vi "Model Initial Values - Main Page.vi"(8 "error in (no error)":errorcluster, 11 "Node Ptr":T1 format="%.0x") -> (0 "error out":errorcluster)   [LabVIEW 2011, in "Model Initial Values Custom Device.lvlib"]
uses:
  Model Initial Values Custom Device.lvlib
  <vilib>/NI Veristand/Custom Device API/Custom Device Item Ref.ctl
  <vilib>/event_ctls.llb/eventvkey.ctl
  <vilib>/NI Veristand/Custom Device API/Custom Device API.lvlib
  Model Initial Values - Global.vi
  <vilib>/NI Veristand/Custom Device Tools/Custom Device Utility Library/Custom Device Utility Library.lvlib
panel:
  in  "Models":i32[](listbox)
  in  "SHDocVw.IWebBrowser2":refnum<k7>(container)
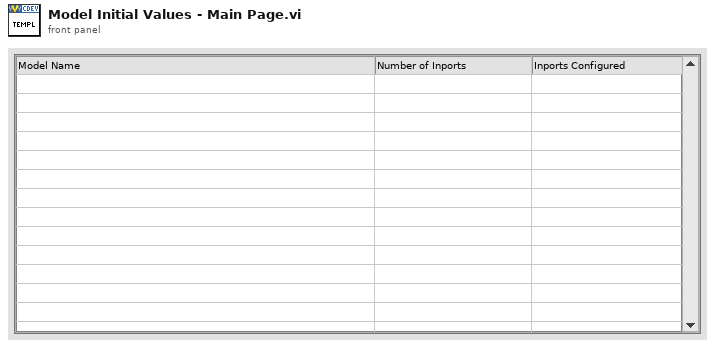
[diagram p1: front panel]
types:
  T1 = typedef "Custom Device API.lvlib/Custom Device Item Ref.ctl" = u64
  T2 = cluster{"Name":string, "Is Channel":bool, "GUID":string}
  T3 = typedef "eventvkey.ctl" = enum16{"ASCII", "Enter", "Return", "Shift", "Ctrl", "Alt", "Cmd", "Opt", "Caps", "NumLock", "Clear", "Break", "Up", "Down", "Left", "Right", "Insert", "Delete", "Home", "End", "PageUp", "PageDown", "Escape", "Help", "Pause", "ScrollLock", "F1", "F2", "F3", "F4", "F5", "F6", "F7", "F8", "F9", "F10", "F11", "F12", "F13", "F14", "F15", "F16", "F17", "F18", "F19", "F20", "F21", "F22", "F23", "F24", "Play", "VolumeUp", "VolumeDown", "Mute", "Two Byte Char"}
  T4 = typedef "Custom Device API.lvlib/Custom Device Commands.ctl" = enum16{"Default", "Item renamed", "Shutdown", "Dynamic button pressed"}
  T5 = enum16{"open", "replace", "create", "open or create", "replace or create", "replace or create with confirmation"}
  T6 = cluster{"MultipleSelection":bool, "ShowCheckBox":bool}
  T7 = typedef "Custom Device API.lvlib/Custom Device Item Info.ctl" = cluster{"Name":string, "Is Channel":bool, "GUID":string}
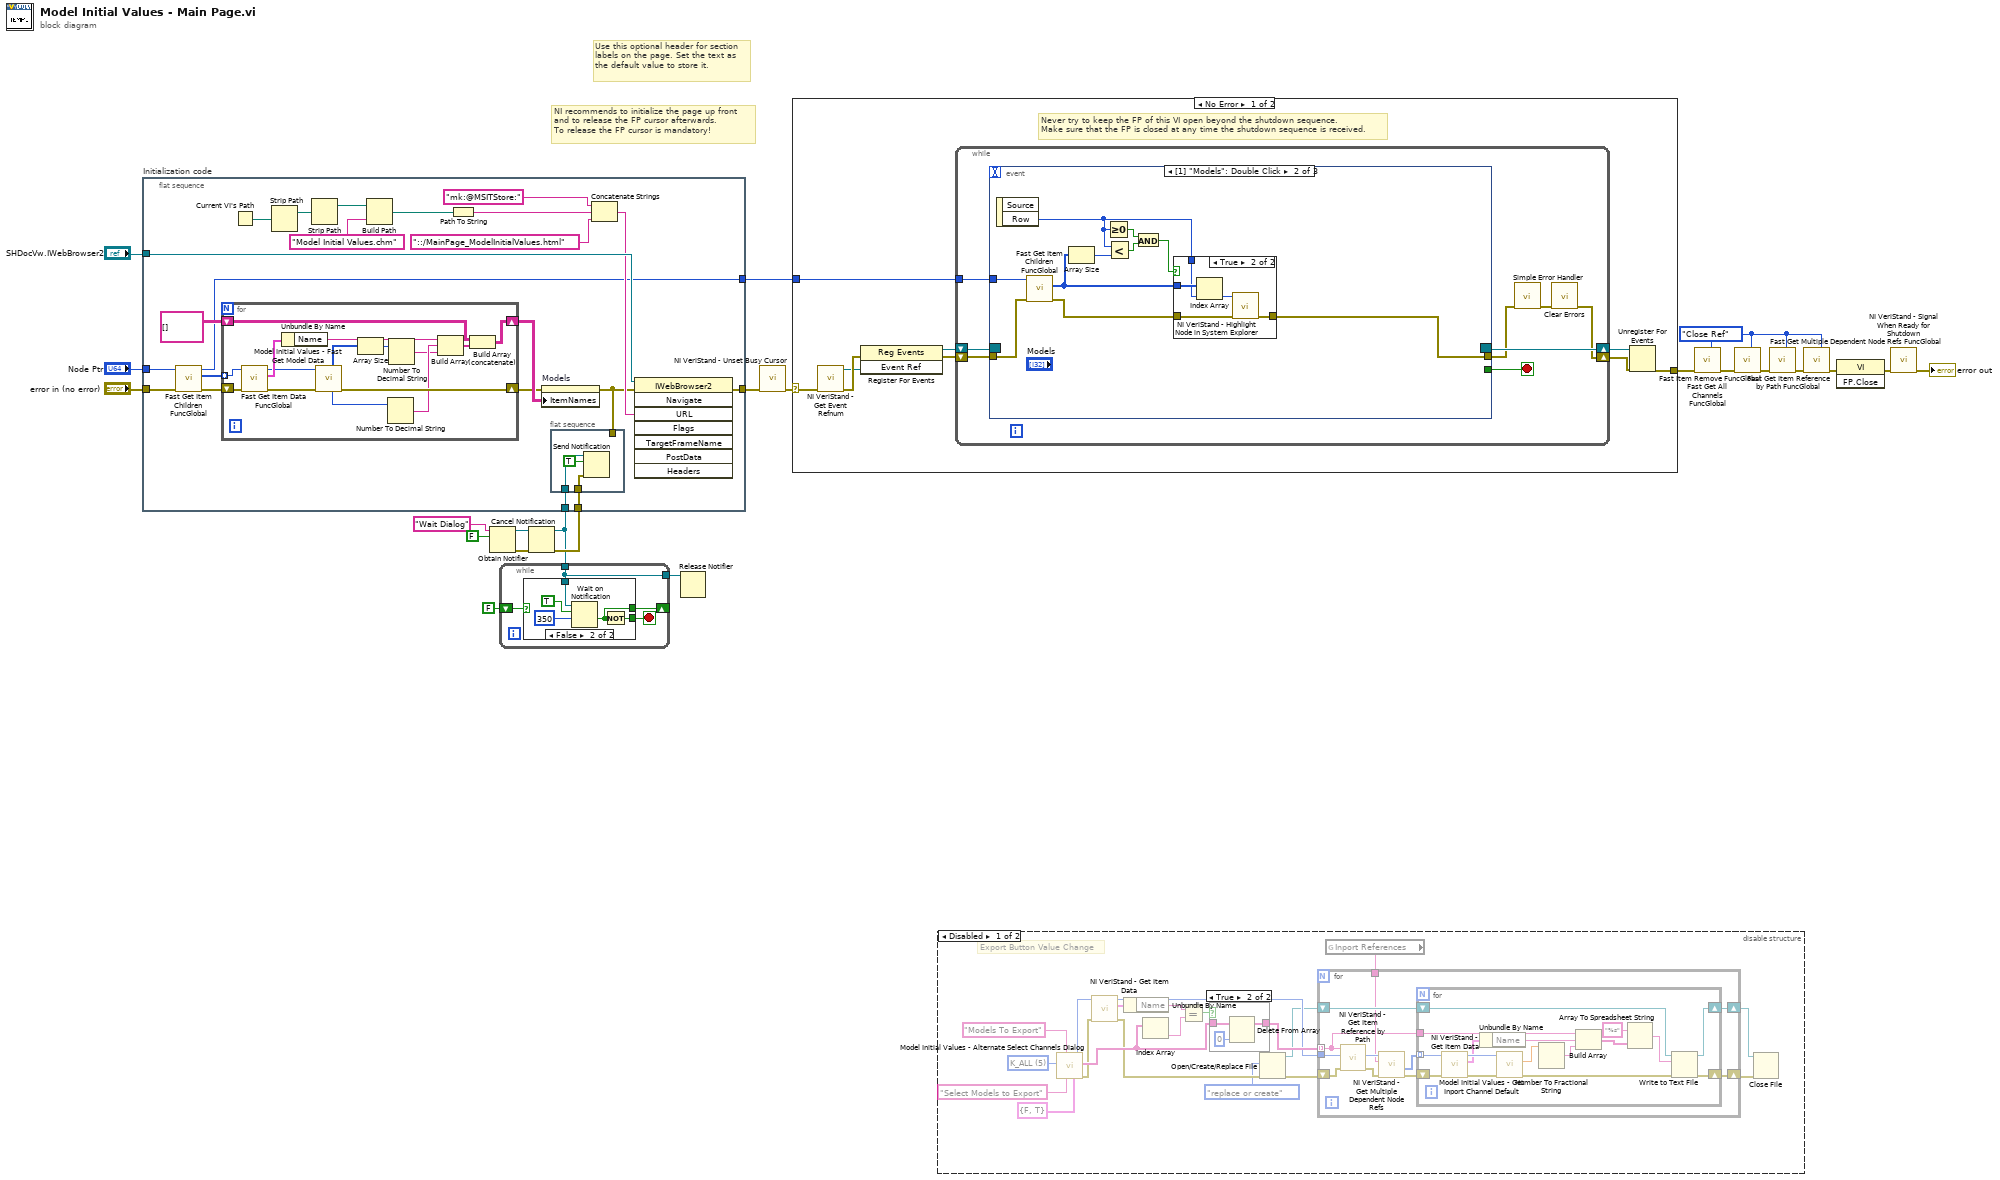
[diagram p0: block diagram]
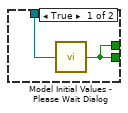
[diagram p2: hidden frame]
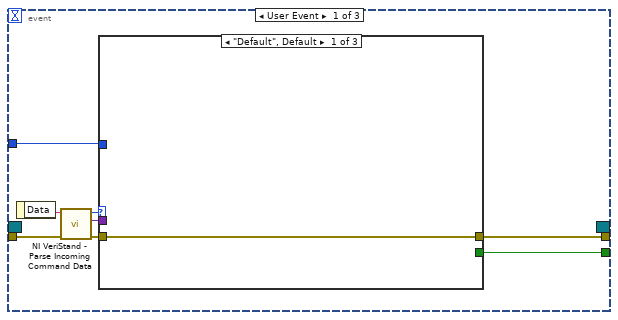
[diagram p5: hidden frame]
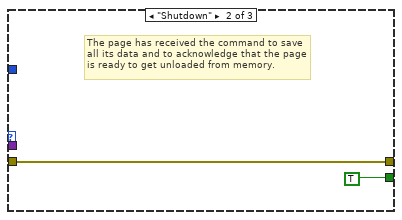
[diagram p6: hidden frame]
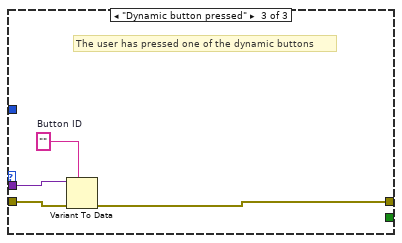
[diagram p7: hidden frame]
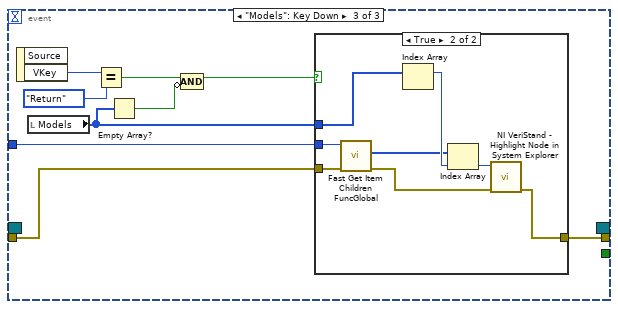
[diagram p9: hidden frame]
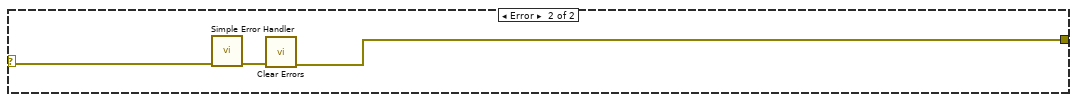
[diagram p11: hidden frame]
diagram:
  w1 = enum16{"Open or Add", "Close Ref"}."Close Ref" ("Action")
  # "Use this optional header for section labels on the page. Set the text as the default value to store it."
  # "NI recommends to initialize the page up front\nand to release the FP cursor afterwards.\nTo release the FP cursor is mandatory!"
  n1 = flat-sequence "Initialization code" {
    tunnel: "error in (no error)" -> [w24]
    tunnel: "Node Ptr" -> [w25]
    tunnel: [w43] -> w20
    tunnel: [w28] -> w17
    tunnel: "SHDocVw.IWebBrowser2" -> [w42]
    tunnel: w4 -> [w27]
    tunnel: w5 -> [w26]
    frame #0 {
      n2 = call "Fast Get Item Children FuncGlobal.vi"("error in (no error)"=w24, "Item Ref in"=w25) -> ("error out"=w30:errorcluster, "Child Refs"=w29:T1[], "Item Ref out"=w28:T1)  [unwired: 6 in, 1 out]
      n3 = for {
        tunnel: w29 -> [w58] mode=indexing
        shift-right: [w61] -> w31
        shift-left: w30 -> [w59]
        shift-right: [w62] -> w44
        shift-left: string[][] [] -> [w60]
        n4 = call "Fast Get Item Data FuncGlobal.vi"("error in (no error)"=w59, "Item Ref in"=w58) -> ("error out"=w49:errorcluster, "Item Info"=w51:T2, "Item Ref out"=w50:T1)  [unwired: 6 in, 1 out]
        n5 = Unbundle By Name(w51) -> ("Name"=w48:string)
        n6 = call "Model Initial Values - Fast Get Model Data.vi"("error in (no error)"=w49, "Local Model Ref in"=w50) -> ("error out"=w61:errorcluster, "Num Inports"=w56:i32, "Inport Refs"=w53:T1[])  [unwired: 4 in, 3 out]
        n7 = Array Size(array=w53) -> (size(s)=w54:i32)
        n8 = Number To Decimal String(number=w56) -> (decimal integer string=w55:string)  [unwired: 1 in]
        n9 = Number To Decimal String(number=w54) -> (decimal integer string=w52:string)  [unwired: 1 in]
        n10 = Build Array(w48, w55, w52) -> (w57:string[])
        n11 = Build Array (concatenate)(w60, w57) -> (w62:string[][])
      }
      n12 = Current VI's Path() -> (path=w33:path)
      n13 = Strip Path(path=w33) -> (stripped path=w34:path)  [unwired: 1 out]
      n14 = Strip Path(path=w34) -> (stripped path=w41:path)  [unwired: 1 out]
      n15 = Build Path(base path=w41, name or relative path="Model Initial Values.chm") -> (appended path=w39:path)
      n16 = Path To String(path=w39) -> (string=w38:string)
      n17 = property on="Models" class="MCListbox (strict)"(error in=w31, "ItemNames"=w44) -> (error out=w23:errorcluster)  [unwired: 1 in, 1 out]
      n18 = flat-sequence {
        tunnel: w27 -> [w47]
        tunnel: w26 -> [w46]
        tunnel: w23 -> [_]
        frame #0 {
          n19 = Send Notification(notification=TRUE, notifier=w47, error in (no error)=w46) -> ()  [unwired: 2 out]
        }
      }
      n20 = Concatenate Strings("mk:@MSITStore:" ("string"), w38, "::/MainPage_ModelInitialValues.html" ("name or relative path")) -> (w35:string)
      n21 = invoke class="IWebBrowser2" method="Navigate"(reference=w42, error in=w23, "URL"=w35) -> (error out=w43:errorcluster)  [unwired: 5 in, 7 out]
    }
  }
  n22 = Obtain Notifier(name (unnamed)="Wait Dialog", notification data type=FALSE) -> (notifier out=w9:refnum<notifier>, error out=w6:errorcluster)  [unwired: 2 in, 1 out]
  n23 = Cancel Notification(0:w9, 3:w6) -> (8:w4:refnum<notifier>, 11:w5:errorcluster)  [unwired: 1 out]
  n24 = while {
    tunnel: w4 -> [w63]
    shift-right: [w64] -> _
    shift-left: FALSE -> [w65]
    tunnel: [w63] -> w7
    stop <- w66 stop-if-true
    n25 = case shown="False" w65 {
      tunnel: [w67 w71] -> w66
      tunnel: w63 -> [w68 w73]
      tunnel: [w67 w69] -> w64
      frame True {
        n26 = call "Model Initial Values - Please Wait Dialog.vi"("notifier out"=w68) -> ("Boolean"=w67:bool)
      }
      frame False {
        n27 = Wait on Notification(notifier=w73, ignore previous (F)=TRUE, timeout in ms (-1)=350) -> (timed out?=w69:bool)  [unwired: 1 in, 3 out]
        n28 = Not(x=w69) -> (.not. x?=w71:bool)
      }
    }
  }
  n29 = Release Notifier(notifier=w7) -> ()  [unwired: 2 in, 3 out]
  n30 = call <vilib>:"NI VeriStand - Unset Busy Cursor.vi"("error in (no error)"=w20) -> ("error out"=w19:errorcluster)  [unwired: 10 out]
  n31 = case shown="No Error" w19 {
    selector: w19 -> [w74 w142]
    tunnel: [w79 w140] -> w14
    tunnel: w17 -> [w75 _]
    frame No Error {
      # "Never try to keep the FP of this VI open beyond the shutdown sequence.\nMake sure that the FP is closed at any time the shutdown sequence is received."
      n32 = call <vilib>:"NI VeriStand - Get Event Refnum.vi"("error in (no error)"=w74) -> ("error out"=w82:errorcluster, "Event Ref"=w78:refnum<user-event>)  [unwired: 9 out]
      n33 = register-events(error in=w82, w78) -> (reference out=w76:refnum<event-registration>, error out=w77:errorcluster)  [unwired: 1 in]
      n34 = while {
        tunnel: w75 -> [w86]
        shift-right: [w83] -> w80
        shift-left: w77 -> [w89]
        shift-right: [w90] -> w81
        shift-left: w76 -> [w88]
        stop <- w87 stop-if-true
        n35 = event shown="[1] \"Models\": Double Click" {
          selector: w88 -> [_ _ _]
          dyn-events: [_ _ _] -> w90
          timeout: _ -> [_ _ _]
          tunnel: w89 -> [w98 w109 w129]
          tunnel: [w95 _ _] -> w87
          tunnel: [w94 w115 w128] -> w85
          tunnel: w86 -> [w93 w107 w130]
          event User Event {
            n36 = event-data() -> ("Data"=w91:string)  [unwired: 1 out]
            n37 = call <vilib>:"NI VeriStand - Parse Incoming Command Data.vi"("error in (no error)"=w98, "Incoming data"=w91) -> ("error out"=w97:errorcluster, "Outgoing data"=w92:variant, "Action"=w96:T4)  [unwired: 7 out]
            n38 = case shown="\"Default\", Default" w96 {
              tunnel: w97 -> [w99 w100 w105]
              tunnel: [_ TRUE _] -> w95
              tunnel: [w99 w100 w102] -> w94
              tunnel: w93 -> [_ _ _]
              tunnel: w92 -> [_ _ w104]
              frame "Default", Default {
              }
              frame "Shutdown" {
                # "The page has received the command to save all its data and to acknowledge that the page is ready to get unloaded from memory."
              }
              frame "Dynamic button pressed" {
                w103 = ""  # Button ID
                # "The user has pressed one of the dynamic buttons"
                n39 = Variant To Data(error in=w105, type=w103, Variant=w104) -> (error out=w102:errorcluster)  [unwired: 1 out]
              }
            }
          }
          event "Models": Double Click {
            n40 = event-data() -> ("Row"=w114:i32)  [unwired: 2 out]
            n41 = call "Fast Get Item Children FuncGlobal.vi"("error in (no error)"=w109, "Item Ref in"=w107) -> ("error out"=w108:errorcluster, "Child Refs"=w106:T1[])  [unwired: 6 in, 2 out]
            n42 = Array Size(array=w106) -> (size(s)=w113:i32)
            n43 = Greater Or Equal To 0?(x=w114) -> (x >= 0?=w112:bool)
            n44 = Less?(x=w114, y=w113) -> (x < y?=w111:bool)
            n45 = And(x=w112, y=w111) -> (x .and. y?=w110:bool)
            n46 = case shown="True" w110 {
              tunnel: [w116 w121] -> w115
              tunnel: w108 -> [w116 w119]
              tunnel: w106 -> [_ w118]
              tunnel: w114 -> [_ w117]
              frame False {
              }
              frame True {
                n47 = Index Array(array=w118, index=w117) -> (element=w120:T1)
                n48 = call <vilib>:"NI VeriStand - Highlight Node in System Explorer.vi"("error in (no error)"=w119, "Item Ref in"=w120) -> ("error out"=w121:errorcluster)  [unwired: 8 in, 1 out]
              }
            }
          }
          event "Models": Key Down {
            n49 = event-data() -> ("VKey"=w127:T3)  [unwired: 2 out]
            n50 = local read "Models"() -> (w124:i32[])
            n51 = Equal?(x=w127, y=eventvkey."Return") -> (x = y?=w125:bool)
            n52 = Empty Array?(array=w124) -> (empty?=w122:bool)
            n53 = Compound Arithmetic op=AND(w125, invert w122) -> (w123:bool)
            n54 = case shown="True" w123 {
              tunnel: w130 -> [_ w134]
              tunnel: w129 -> [w131 w135]
              tunnel: [w131 w139] -> w128
              tunnel: w124 -> [_ w137]
              frame False {
              }
              frame True {
                n55 = call "Fast Get Item Children FuncGlobal.vi"("error in (no error)"=w135, "Item Ref in"=w134) -> ("error out"=w132:errorcluster, "Child Refs"=w133:T1[])  [unwired: 6 in, 2 out]
                n56 = Index Array(array=w137) -> (element=w138:i32)  [unwired: 1 in]
                n57 = Index Array(array=w133, index=w138) -> (element=w136:T1)
                n58 = call <vilib>:"NI VeriStand - Highlight Node in System Explorer.vi"("error in (no error)"=w132, "Item Ref in"=w136) -> ("error out"=w139:errorcluster)  [unwired: 8 in, 1 out]
              }
            }
          }
        }
        n59 = call <vilib>:"Simple Error Handler.vi"("error in (no error)"=w85) -> ("error out"=w84:errorcluster)  [unwired: 1 in, 7 out]
        n60 = call <vilib>:"Clear Errors.vi"("error in (no error)"=w84) -> ("error out"=w83:errorcluster)  [unwired: 6 out]
      }
      n61 = Unregister For Events(event registration refnum=w81, error in=w80) -> (error out=w79:errorcluster)
    }
    frame Error {
      n62 = call <vilib>:"Simple Error Handler.vi"("error in (no error)"=w142) -> ("error out"=w141:errorcluster)  [unwired: 1 in, 7 out]
      n63 = call <vilib>:"Clear Errors.vi"("error in (no error)"=w141) -> ("error out"=w140:errorcluster)  [unwired: 6 out]
    }
  }
  n64 = disable-structure shown="Disabled" {
    frame Disabled {
      w144 = u8 5 items=["K_CHAN_R", "K_CHAN_W", "K_CHAN_RW", "K_CHAN_VOLT", "K_CHAN_FAULT", "K_ALL", "K_CUSTOM"] ("Filter")
      # "Export Button Value Change"
      n65 = call "Model Initial Values - Alternate Select Channels Dialog.vi"("Selection Properties"=T6 {"MultipleSelection"=FALSE, "ShowCheckBox"=TRUE}, "FP Win Title"="Select Models to Export", "Channel Label"="Models To Export", "Filter"=w144) -> ("error out"=w158:errorcluster, "Channel Names"=w161:string[], "Start Item Ref"=w154:T1)  [unwired: 3 in, 2 out]
      n66 = call <vilib>:"NI VeriStand - Get Item Data.vi"("error in (no error)"=w158, "Item Ref in"=w154) -> ("error out"=w159:errorcluster, "Item Info"=w153:T7, "Item Ref out"=w155:T1)  [unwired: 6 in, 1 out]
      n67 = Unbundle By Name(w153) -> ("Name"=w156:string)
      n68 = Index Array(array=w161) -> (element=w157:string)  [unwired: 1 in]
      n69 = Equal?(x=w156, y=w157) -> (x = y?=w160:bool)
      n70 = case shown="True" w160 {
        tunnel: w161 -> [w163 w166]
        tunnel: [w163 w164] -> w162
        frame False {
        }
        frame True {
          n71 = Delete From Array(array=w166, index=0) -> (array with subset deleted=w164:string[])  [unwired: 1 in, 1 out]
        }
      }
      n72 = Open/Create/Replace File(error in=w159, operation (0:open)=T5."replace or create") -> (refnum out=w149:refnum<file>, error out=w147:errorcluster)  [unwired: 4 in, 1 out]
      n73 = global read "Model Initial Values - Global.vi" "Inport References"() -> (w150:string)
      n74 = for {
        tunnel: w162 -> [w167] mode=indexing
        shift-right: [w177] -> w152
        shift-left: w149 -> [w176]
        shift-right: [w175] -> w151
        shift-left: w147 -> [w173]
        tunnel: w155 -> [w174]
        tunnel: w150 -> [w171]
        n75 = call <vilib>:"NI VeriStand - Get Item Reference by Path.vi"("error in (no error)"=w173, "Root Ref"=w174, "Item Path in"=w167) -> ("error out"=w170:errorcluster, "Item Ref"=w172:T1)  [unwired: 5 in, 2 out]
        n76 = call <vilib>:"NI VeriStand - Get Multiple Dependent Node Refs.vi"("error in (no error)"=w170, "Base Property Name"=w171, "Item Ref in"=w172) -> ("error out"=w168:errorcluster, "Dependent Node Refs"=w169:T1[])  [unwired: 6 in, 1 out]
        n77 = for {
          shift-right: [w193] -> w175
          shift-left: w168 -> [w181]
          shift-right: [w189] -> w177
          shift-left: w176 -> [w190]
          tunnel: w169 -> [w178] mode=indexing
          tunnel: w167 -> [w179]
          n78 = call <vilib>:"NI VeriStand - Get Item Data.vi"("error in (no error)"=w181, "Item Ref in"=w178) -> ("error out"=w186:errorcluster, "Item Info"=w183:T7, "Item Ref out"=w185:T1)  [unwired: 6 in, 1 out]
          n79 = Unbundle By Name(w183) -> ("Name"=w184:string)
          n80 = call "Model Initial Values - Get Inport Channel Default.vi"("error in"=w186, "Item Ref in"=w185) -> ("error out"=w182:errorcluster, "Default Value"=w187:dbl)  [unwired: 6 in, 1 out]
          n81 = Number To Fractional String(number=w187) -> (F-format string=w188:string)  [unwired: 3 in]
          n82 = Build Array(w179, w184, w188) -> (w180:string[])
          n83 = Array To Spreadsheet String(array=w180, 3:"%s" ("format string")) -> (spreadsheet string=w191:string)  [unwired: 1 in]
          n84 = Write to Text File(file (use dialog)=w190, text=w191, error in=w182) -> (refnum out=w189:refnum<file>, error out=w193:errorcluster)  [unwired: 1 in, 1 out]
        }
      }
      n85 = Close File(refnum=w152, error in=w151) -> ()  [unwired: 2 out]
    }
    frame Enabled {
    }
  }
  n86 = call "Fast Get All Channels FuncGlobal.vi"("Action"=w1, "error in"=w14) -> ("error out"=w13:errorcluster)  [unwired: 6 in, 3 out]
  n87 = call "Fast Item Remove FuncGlobal.vi"("Action"=w1, "error in (no error)"=w13) -> ("error out"=w12:errorcluster)  [unwired: 8 in, 1 out]
  n88 = call "Fast Get Multiple Dependent Node Refs FuncGlobal.vi"("Action"=w1, "error in (no error)"=w12) -> ("error out"=w3:errorcluster)  [unwired: 7 in, 2 out]
  n89 = call "Fast Get Item Reference by Path FuncGlobal.vi"("Action"=w1, "error in (no error)"=w3) -> ("error out"=w2:errorcluster)  [unwired: 6 in, 3 out]
  n90 = invoke class="VI" method="FP.Close"(error in=w2) -> (error out=w22:errorcluster)  [unwired: 2 in, 2 out]
  n91 = call <vilib>:"NI VeriStand - Signal When Ready for Shutdown.vi"("error in (no error)"=w22) -> ("error out"=→"error out":errorcluster)  [unwired: 10 out]
